vi "iRobot Navigation Target.vi"() -> ()   [LabVIEW 2015]
uses:
  iRobot/Sensor/OI Mode.ctl
  iRobot/Sensor/Charging Sources Available.ctl
  iRobot/Sensor/Cargo Bay Digital Inputs.ctl
  iRobot/Sensor/Charging State.ctl
  iRobot/Sensor/Buttons.ctl
  iRobot/Sensor/Low-Side Driver + Wheel Overcurrent.ctl
  iRobot/Sensor/Bumps + Wheel Drops.ctl
  <vilib>/Statechart/Infrastructure/RTStatechart/RunTime SCN.xnode
  iRobot/Sensor/Sensor Group 6.ctl
  Accelerometer.ctl
  iRobot Navigation State Machine.lvsc
  iRobot Navigation State Machine.lvsc/Inputs.ctl
  iRobot Navigation State Machine.lvsc/Outputs.ctl
  iRobot Navigation State Machine.lvsc/Trigger.ctl
  iRobot Navigation State Machine.lvsc/State.ctl
  iRobot Navigation State Machine.lvsc/StatechartState.ctl
  <vilib>/myRIO/Instrument Drivers/Utilities/Utilities.lvlib
  iRobot Sensors.ctl
panel:
  out "temp ind.":dbl[](array[numeric])
  in  "Barcode Time Threshold":dbl
  in  "Barcode Threshold":dbl
  in  "Tab Control":T1(tab)
  out "iRobot Sensors (graphical)":T2 {"Right Wheel (mm/s)" scale=-500.0..500.0; "Left Wheel (mm/s)" scale=-500.0..500.0}
  out "Active States":T4
  out "error out":errorcluster
  in  "Wheel Speed (mm/s)":i16(slide)=100 scale=0.0..500.0
  in  "accel smoothing (0-1)":dbl=0.1
  in  "stop":bool
  out "Target Running":bool
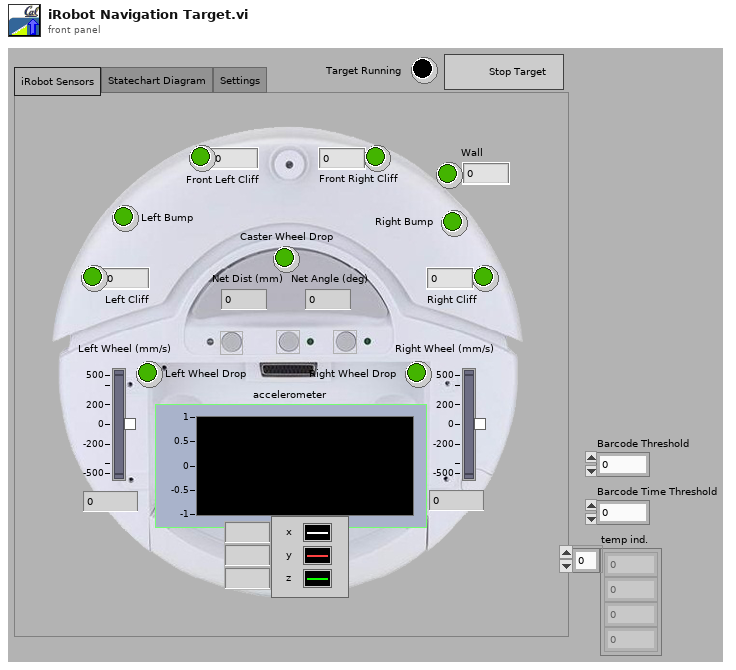
[diagram p1: front panel]
types:
  T1 = enum32{"iRobot Sensors", "Statechart Diagram", "Settings"}
  T2 = typedef "iRobot Sensors.ctl" = cluster{"Caster Wheel Drop":bool, "Left Wheel Drop":bool, "Right Wheel Drop":bool, "Left Bump":bool, "Right Bump":bool, "Left Cliff":bool, "Front Left Cliff":bool, "Front Right Cliff":bool, "Right Cliff":bool, "Wall":bool, "Net Dist (mm)":i32, "Net Angle (deg)":i32, "Wall":u16, "Left Cliff":u16, "Front Left Cliff":u16, "Front Right Cliff":u16, "Right Cliff":u16, "Left Wheel (mm/s)":i16, "Right Wheel (mm/s)":i16, "accelerometer":T3}
  T3 = typedef "Accelerometer.ctl" = cluster{"x axis (g)":dbl, "y axis (g)":dbl, "z axis (g)":dbl}
  T4 = typedef "iRobot Navigation State Machine.lvsc/StatechartState.ctl" = T5[]
  T5 = typedef "iRobot Navigation State Machine.lvsc/State.ctl" = enum16{"NI.SC.Initial", "NI.SC.History", "NI.SC.ShallowHistory", "NI.SC.Terminal", "Pause", "Run", "Pause\\Detect Play Button\\Pause;\nWait for\nbutton\nrelease", "Pause\\Detect Play Button\\Unpause;\nwait for\nbutton release", "Pause\\Detect Play Button\\Unpause;\nwait for\nbutton press", "Run\\Detect Obstacles\\Stop", "Run\\Detect Obstacles\\Speed Up", "Run\\Detect Obstacles\\Turn Right", "Run\\Detect Obstacles\\Turn Left", "Run\\Detect Obstacles\\Light", "Run\\Detect Obstacles\\Dark", "Run\\Detect Obstacles\\Drive"}
  T6 = typedef "iRobot UART Port Type.ctl" = refnum<visa-resource-name>
  T7 = typedef "iRobot Navigation State Machine.lvsc/Inputs.ctl" = cluster{"net distance (mm)":i32, "net angle (deg)":i32, "Max Wheel Speed (mm/s)":i16, "accelerometer":T3, "iRobot Sensors":T8, "Is Simulator?":bool, "Barcode Sensor Threshold":dbl, "Barcode Time Threshold":dbl}
  T8 = typedef "Sensor Group 6.ctl" = cluster{"Bumps + Wheel Drops":T9, "Wall":bool, "Cliff Left":bool, "Cliff Front Left":bool, "Cliff Front Right":bool, "Cliff Right":bool, "Virtual Wall":bool, "Low-Side Driver + Wheel Overcurrent":T10, "Infrared":u8, "Buttons":T11, "Distance (mm)":i32, "Angle (deg)":i32, "Charging State":T12, "Voltage (mV)":u16, "Current (mA)":i16, "Battery Temperature (deg C)":i8, "Battery Charge (mAh)":u16, "Battery Capacity (mAh)":u16, "Wall Signal (0-4095)":u16, "Cliff Left Signal (0-4095)":u16, "Cliff Front Left Signal (0-4095)":u16, "Cliff Front Right Signal (0-4095)":u16, "Cliff Right Signal (0-4095)":u16, "Cargo Bay Digital Inputs":T13, "Cargo Bay Analog Signal (0-1023)":u16, "Charging Sources Available":T14, "OI Mode":T15, "Song Number":u8, "Song Playing":bool, "Number of Stream Packets":u8, "Requested Velocity (mm/s)":i16, "Requested Radius (mm)":i16, "Requested Right Wheel Velocity (mm/s)":i16, "Requested Left Wheel Velocity (mm/s)":i16}
  T9 = typedef "Bumps + Wheel Drops.ctl" = cluster{"Wheeldrop Caster":bool, "Wheeldrop Left":bool, "Wheeldrop Right":bool, "Bump Left":bool, "Bump Right":bool}
  T10 = typedef "Low-Side Driver + Wheel Overcurrent.ctl" = cluster{"Low-Side Driver 0":bool, "Low-Side Driver 1":bool, "Low-Side Driver 2":bool, "Left Wheel":bool, "Right Wheel":bool}
  T11 = typedef "Buttons.ctl" = cluster{"Advance":bool, "Play":bool}
  T12 = typedef "Charging State.ctl" = enum16{"Not Charging", "Reconditioning Charging", "Full Charging", "Trickle Charging", "Waiting", "Charging Fault Condition"}
  T13 = typedef "Cargo Bay Digital Inputs.ctl" = cluster{"Digital Input 0":bool, "Digital Input 1":bool, "Digital Input 2":bool, "Digital Input 3":bool, "Device Detect":bool}
  T14 = typedef "Charging Sources Available.ctl" = cluster{"Internal Charger":bool, "Home Base":bool}
  T15 = typedef "OI Mode.ctl" = enum16{"Off", "Passive", "Safe", "Full"}
  T16 = typedef "iRobot Navigation State Machine.lvsc/Outputs.ctl" = cluster{"Left Wheel Speed (mm/s)":i16, "Right Wheel Speed (mm/s)":i16, "Array":dbl[]}
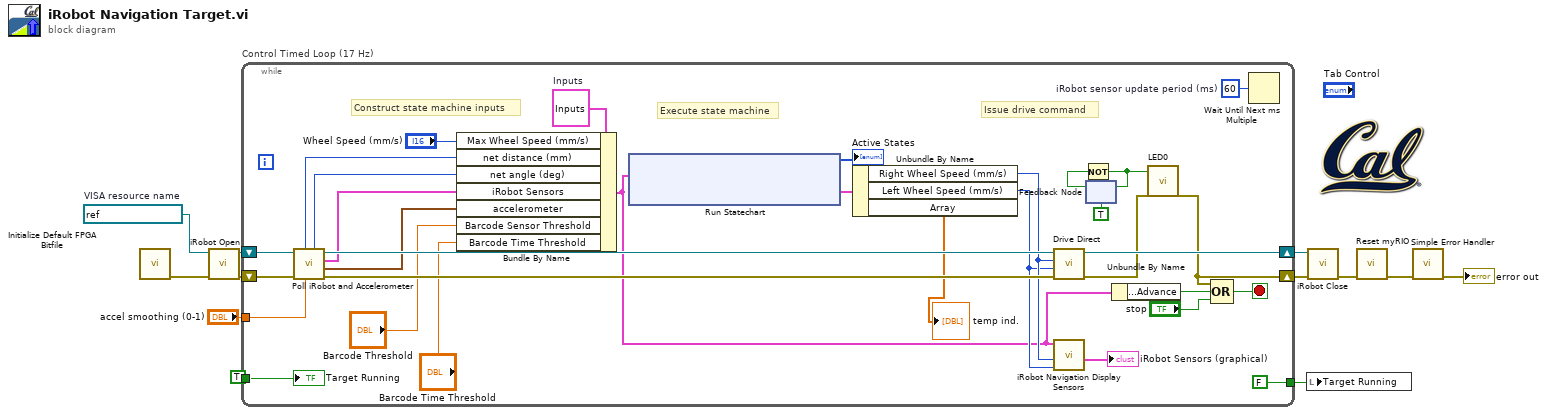
[diagram p0: block diagram]
diagram:
  w6 = refnum<visa-resource-name> "ASRL1::INSTR"  # VISA resource name
  n1 = call <vilib>:"Initialize Default FPGA Bitfile.vi"() -> ("error out"=w4:errorcluster)  [unwired: 11 in]
  n2 = call "iRobot Open.vi"("error in (no error)"=w4, "UART port in"=w6) -> ("error out"=w11:errorcluster, "UART port out"=w10:T6)  [unwired: 8 in]
  n3 = while "Control Timed Loop (17 Hz)" {
    shift-right: [w44] -> w12
    shift-left: w10 -> [w39]
    shift-right: [w26] -> w7
    shift-left: w11 -> [w38]
    tunnel: TRUE ("stop") -> [w32]
    tunnel: [FALSE ("stop")] -> w8
    tunnel: "accel smoothing (0-1)" -> [w18]
    stop <- w43 stop-if-true
    w16 = u32 60  # iRobot sensor update period (ms)
    w41 = T7 {"net distance (mm)"=0, "net angle (deg)"=0, "Max Wheel Speed (mm/s)"=0, "accelerometer"={"x axis (g)"=0.0, "y axis (g)"=0.0, "z axis (g)"=0.0}, "iRobot Sensors"={"Bumps + Wheel Drops"={"Wheeldrop Caster"=FALSE, "Wheeldrop Left"=FALSE, "Wheeldrop Right"=FALSE, "Bump Left"=FALSE, "Bump Right"=FALSE}, "Wall"=FALSE, "Cliff Left"=FALSE, "Cliff Front Left"=FALSE, "Cliff Front Right"=FALSE, "Cliff Right"=FALSE, "Virtual Wall"=FALSE, "Low-Side Driver + Wheel Overcurrent"={"Low-Side Driver 0"=FALSE, "Low-Side Driver 1"=FALSE, "Low-Side Driver 2"=FALSE, "Left Wheel"=FALSE, "Right Wheel"=FALSE}, "Infrared"=255, "Buttons"={"Advance"=FALSE, "Play"=FALSE}, "Distance (mm)"=0, "Angle (deg)"=0, "Charging State"=enum."Not Charging", "Voltage (mV)"=0, "Current (mA)"=0, "Battery Temperature (deg C)"=0, "Battery Charge (mAh)"=0, "Battery Capacity (mAh)"=0, "Wall Signal (0-4095)"=0, "Cliff Left Signal (0-4095)"=0, "Cliff Front Left Signal (0-4095)"=0, "Cliff Front Right Signal (0-4095)"=0, "Cliff Right Signal (0-4095)"=0, "Cargo Bay Digital Inputs"={"Digital Input 0"=FALSE, "Digital Input 1"=FALSE, "Digital Input 2"=FALSE, "Digital Input 3"=FALSE, "Device Detect"=FALSE}, "Cargo Bay Analog Signal (0-1023)"=0, "Charging Sources Available"={"Internal Charger"=FALSE, "Home Base"=FALSE}, "OI Mode"=enum."Off", "Song Number"=0, "Song Playing"=FALSE, "Number of Stream Packets"=0, "Requested Velocity (mm/s)"=0, "Requested Radius (mm)"=0, "Requested Right Wheel Velocity (mm/s)"=0, "Requested Left Wheel Velocity (mm/s)"=0}, "Is Simulator?"=FALSE, "Barcode Sensor Threshold"=0.0, "Barcode Time Threshold"=0.0}  # Inputs
    # "Issue drive command"
    # "Execute state machine"
    # "Construct state machine inputs"
    n4 = call "Poll iRobot and Accelerometer.vi"("accel smoothing (0-1)"=w18, "error in"=w38, "UART port in"=w39) -> ("error out"=w37:errorcluster, "Acceleration (g)"=w17:T3, "iRobot SensorGroup6"=w25:T8, "UART port out"=w36:T6, "net angle (deg)"=w34:i32, "net distance (mm)"=w35:i32)  [unwired: 3 in]
    n5 = Bundle By Name(cluster=w41, "Max Wheel Speed (mm/s)"="Wheel Speed (mm/s)", "net distance (mm)"=w35, "net angle (deg)"=w34, "iRobot Sensors"=w25, "accelerometer"=w17, "Barcode Sensor Threshold"="Barcode Threshold", "Barcode Time Threshold"="Barcode Time Threshold") -> (w20:T7)
    n6 = xnode "Run Statechart"("Inputs"=w20) -> ("Outputs"=w42:T16, "Active States"=→"Active States":T4)  [unwired: 2 in, 1 out]
    n7 = Unbundle By Name(w42) -> ("Right Wheel Speed (mm/s)"=w23:i16, "Left Wheel Speed (mm/s)"=w22:i16, "Array"=→"temp ind.":dbl[])
    n8 = call "Drive Direct.vi"("error in"=w37, "Left Wheel Velocity (mm/s)"=w22, "Right Wheel Velocity (mm/s)"=w23, "UART port in"=w36) -> ("error out"=w27:errorcluster, "UART port out"=w44:T6)  [unwired: 6 in]
    n9 = call "iRobot Navigation Display Sensors.vi"("Left Wheel (mm/s)"=w22, "Right Wheel (mm/s)"=w23, "Statechart Inputs"=w20) -> ("iRobot Sensors (graphical)"=→"iRobot Sensors (graphical)":T2)  [unwired: 6 in]
    n10 = feedback #1(TRUE) -> (w28:bool)
    n11 = Not(x=w28) -> (.not. x?=w29:bool)
    n12 = feedback-in #1(w29) -> ()
    n13 = Unbundle By Name(w20) -> ("iRobot Sensors.Buttons.Advance"=w19:bool)
    n14 = call "LED0"("LED0"=w29, "error in (no error)"=w27) -> ("error out"=w26:errorcluster)  [unwired: 25 in]
    n15 = Compound Arithmetic op=OR(w26, w19, "stop") -> (w43:bool)
    n16 = Wait Until Next ms Multiple(millisecond multiple=w16) -> ()  [unwired: 1 out]
    "Target Running" <- w32
  }
  n17 = local write "Target Running"(w8) -> ()
  n18 = call "iRobot Close.vi"("error in"=w7, "UART port in"=w12) -> ("error out"=w1:errorcluster)  [unwired: 9 in]
  n19 = call <vilib>:"Reset myRIO.vi"("error in (no error)"=w1) -> ("error out"=w5:errorcluster)  [unwired: 10 in]
  n20 = call <vilib>:"Simple Error Handler.vi"("error in (no error)"=w5) -> ("error out"=→"error out":errorcluster)  [unwired: 4 in, 4 out]
